vi "FFT_Alpha_Beta_Power_Extractor.vi"(11 "EEG_Signal":dbl[](array[numeric])) -> (2 "Beta":dbl, 3 "Alpha":dbl)   [LabVIEW 2014]
uses:
  <vilib>/gmath/NI_Gmath.lvlib
  <vilib>/Analysis/NI_AALPro.lvlib
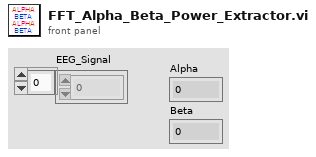
[diagram p1: front panel]
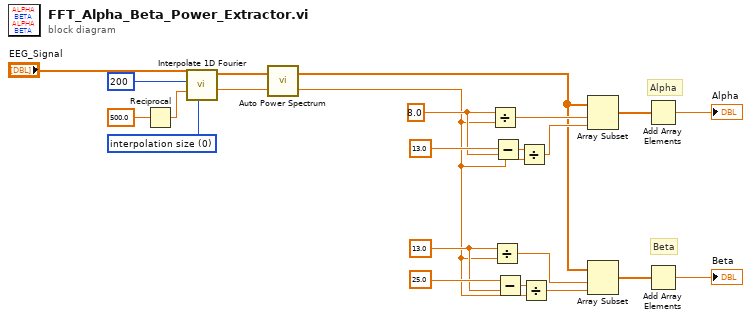
[diagram p0: block diagram]
diagram:
  w11 = 13.0 ("x")
  w14 = 8.0 ("x")
  w20 = u16 0 items=["interpolation size", "interpolation factor"] ("type")
  # "Beta"
  # "Alpha"
  n1 = Reciprocal(x=500.0 ("Resampling(Hz)")) -> (1/x=w22:dbl)
  n2 = call <vilib>:"Interpolate 1D Fourier.vi"("type"=w20, "dt in"=w22, "n"=200, "X"="EEG_Signal") -> ("dt out"=w17:dbl, "Y"=w18:dbl[])  [unwired: 4 in, 2 out]
  n3 = call <vilib>:"Auto Power Spectrum.vi"("dt"=w17, "Signal (V)"=w18) -> ("df"=w10:dbl, "Power Spectrum (V^2 rms)"=w5:dbl[])
  n4 = Divide(x=w14, y=w10) -> (x/y=w9:dbl)
  n5 = Divide(x=w11, y=w10) -> (x/y=w6:dbl)
  n6 = Subtract(x=13.0, y=w14) -> (x-y=w16:dbl)
  n7 = Subtract(x=25.0, y=w11) -> (x-y=w13:dbl)
  n8 = Divide(x=w16, y=w10) -> (x/y=w8:dbl)
  n9 = Divide(x=w13, y=w10) -> (x/y=w7:dbl)
  n10 = Array Subset(array=w5, index=w9, length=w8) -> (w4:dbl[])
  n11 = Array Subset(array=w5, index=w6, length=w7) -> (w3:dbl[])
  n12 = Add Array Elements(numeric array=w4) -> (sum=→"Alpha":dbl)
  n13 = Add Array Elements(numeric array=w3) -> (sum=→"Beta":dbl)
